vi "UMLEditor_GetP.vi"(8 "error in (no error)":errorcluster, 10 "GetProjectRefByName/or Ref":variant) -> (0 "error out":errorcluster, 1 "j":i32, 2 "i":i32, 3 "ClassesNamesAndPaths":T1[](array[typedef]), 4 "A":i32, 6 "B":i32)   [LabVIEW 2012]
uses:
  <resource>/Framework/Providers/Open_GDS/ClassProviders/Common/CommonVIs/CommonVIs_ClassNamePathType.ctl
  <resource>/Framework/Providers/Open_GDS/ClassProviders/Common/LvClass_class/GDSLvClass_ClassTypeSettingNames.ctl
  <resource>/Framework/Providers/Open_GDS/ClassProviders/Provider_EndevoGOOP300/EndevoProviderName.ctl
  <resource>/Framework/Providers/Open_GDS/ClassProviders/Provider_EndevoGOOP400/EndevoG4ProviderName.ctl
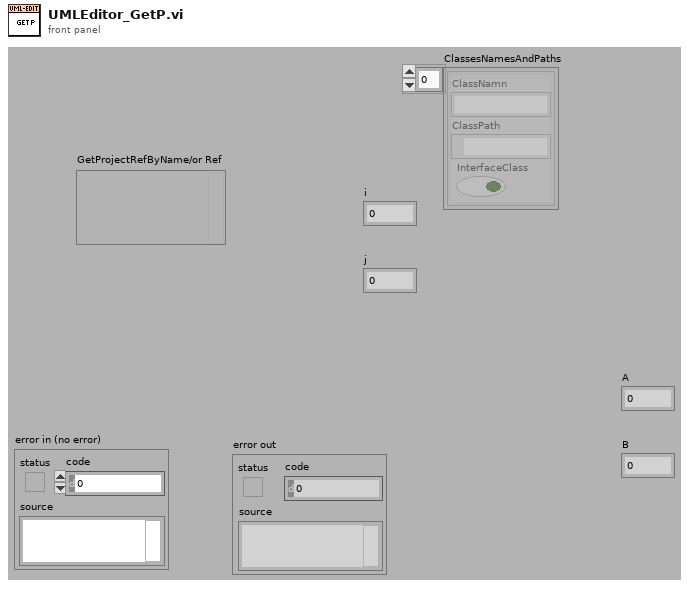
[diagram p1: front panel]
types:
  T1 = typedef "CommonVIs_ClassNamePathType.ctl" = cluster{"ClassNamn":string, "ClassPath":path, "InterfaceClass":bool}
  T2 = typedef "EndevoG4ProviderName.ctl" = enum16{"EndevoGOOP400"}
  T3 = typedef "EndevoProviderName.ctl" = enum16{"EndevoGOOP300"}
  T4 = typedef "GDSLvClass_ClassTypeSettingNames.ctl" = enum16{"EndevoGOOP_ClassProvider", "EndevoGOOP_TemplateUsed", "EndevoGOOP_TemplateVersion", "EndevoGOOP_PlugIns", "EndevoGOOP_ConnectorPanePattern"}
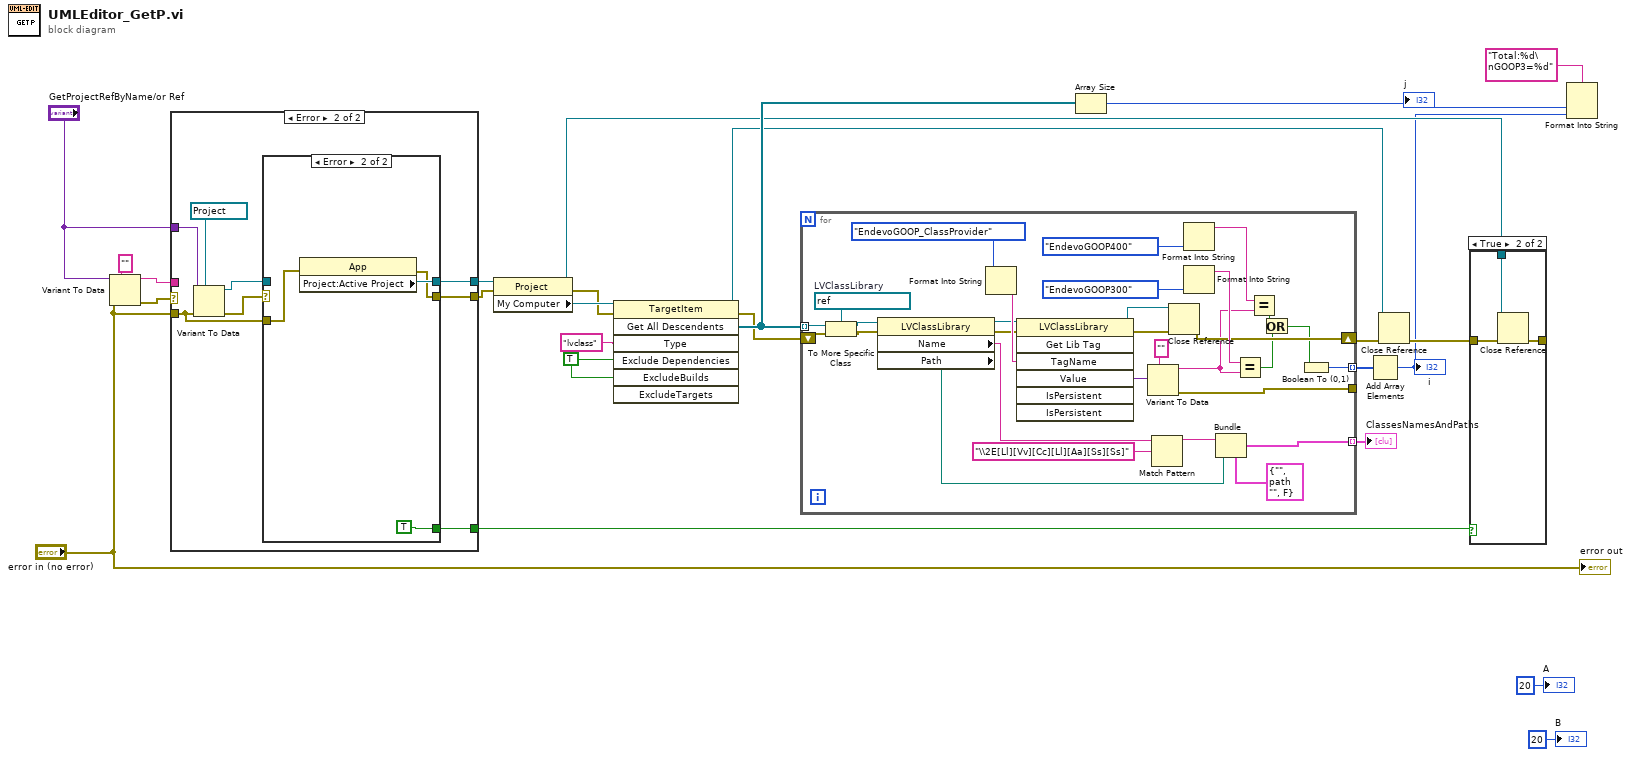
[diagram p0: block diagram]
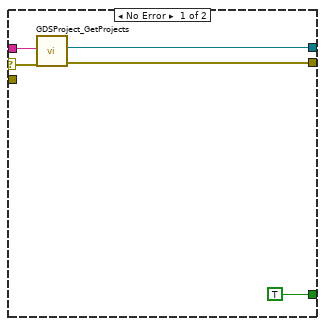
[diagram p3: hidden frame]
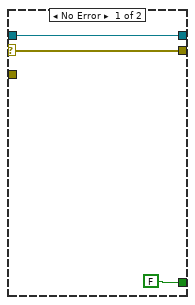
[diagram p4: hidden frame]
diagram:
  w4 = TRUE ("ExcludeDependencies")
  n1 = Variant To Data(error in="error in (no error)", type="", Variant="GetProjectRefByName/or Ref") -> (data=w15:string, error out=w14:errorcluster)
  n2 = case shown="Error" w14 {
    selector: w14 -> [w27 _]
    tunnel: [w30 w34] -> w25
    tunnel: [w29 w33] -> w21
    tunnel: w15 -> [w28 _]
    tunnel: "error in (no error)" -> [_ w32]
    tunnel: "GetProjectRefByName/or Ref" -> [_ w37]
    tunnel: [TRUE w31] -> w5
    frame No Error {
      n3 = call <resource>:"GDSProject_GetProjects.vi"("GetProjectRefByName"=w28, "error in (no error)"=w27) -> ("Project Refnum"=w30:refnum<vi>, "error out"=w29:errorcluster)  [unwired: 1 in, 15 out]
    }
    frame Error {
      n4 = Variant To Data(error in=w32, type=refnum<vi> refnum ("Project Refnum"), Variant=w37) -> (data=w35:refnum<vi>, error out=w36:errorcluster)
      n5 = case shown="Error" w36 {
        selector: w36 -> [w40 _]
        tunnel: w35 -> [w41 _]
        tunnel: [w41 w45] -> w34
        tunnel: [w40 w43] -> w33
        tunnel: w32 -> [_ w44]
        tunnel: [FALSE TRUE] -> w31
        frame No Error {
        }
        frame Error {
          n6 = property class="App"(error in=w44) -> (error out=w43:errorcluster, "Project:Active Project"=w45:refnum<vi>)  [unwired: 1 in, 1 out]
        }
      }
    }
  }
  n7 = property class="Project"(reference=w25, error in=w21) -> (reference out=w17:refnum<vi>, error out=w12:errorcluster, "My Computer"=w24:refnum<vi>)
  n8 = invoke class="TargetItem" method="Get All Descendents"(reference=w24, error in=w12, "Type"="lvclass", "Exclude Dependencies"=w4, "ExcludeBuilds"=w4) -> (reference out=w18:refnum<vi>, error out=w11:errorcluster, "All Descendents"=w20:refnum<vi>[])  [unwired: 2 in, 4 out]
  n9 = for {
    tunnel: w20 -> [w70] mode=indexing
    tunnel: [w67] -> w22 mode=indexing
    shift-right: [w63] -> w19
    shift-left: w11 -> [w66]
    tunnel: [w62] -> _
    tunnel: [w53] -> w3 mode=indexing
    w75 = refnum<vi> refnum  # LVClassLibrary
    n10 = To More Specific Class(target class=w75, reference=w70, error in=w66) -> (specific class reference=w61:refnum<vi>, error out=w60:errorcluster)
    n11 = property class="LVClassLibrary"(reference=w61, error in=w60) -> (reference out=w59:refnum<vi>, error out=w58:errorcluster, "Name"=w57:string, "Path"=w54:path)
    n12 = Format Into String(GDSLvClass_ClassTypeSettingNames."EndevoGOOP_ClassProvider" ("ClassTypeSettingNames")) -> (resulting string=w72:string)  [unwired: 3 in, 1 out]
    n13 = invoke class="LVClassLibrary" method="Get Lib Tag"(reference=w59, error in=w58, "TagName"=w72) -> (reference out=w65:refnum<vi>, error out=w64:errorcluster, "Value"=w74:variant)  [unwired: 4 in, 4 out]
    n14 = Variant To Data(type="", Variant=w74) -> (data=w51:string, error out=w62:errorcluster)  [unwired: 1 in]
    n15 = Match Pattern(string=w57, regular expression="\\2E[Ll][Vv][Cc][Ll][Aa][Ss][Ss]") -> (before substring=w55:string)  [unwired: 4 out]
    n16 = Close Reference(reference=w65, error in (no error)=w64) -> (error out=w63:errorcluster)
    n17 = Format Into String(EndevoG4ProviderName."EndevoGOOP400" ("ProviderName")) -> (resulting string=w50:string)  [unwired: 3 in, 1 out]
    n18 = Format Into String(EndevoProviderName."EndevoGOOP300" ("ProviderName")) -> (resulting string=w68:string)  [unwired: 3 in, 1 out]
    n19 = Bundle(cluster=T1 {"ClassNamn"="", "ClassPath"=path "", "InterfaceClass"=FALSE} ("Cluster"), "ClassNamn"=w55, "ClassPath"=w54) -> (w53:T1)  [unwired: 1 in]
    n20 = Equal?(x=w68, y=w51) -> (x = y?=w48:bool)
    n21 = Equal?(x=w50, y=w51) -> (x = y?=w49:bool)
    n22 = Or(x=w49, y=w48) -> (x .or. y?=w47:bool)
    n23 = Boolean To (0,1)(Boolean=w47) -> (0, 1=w67:i16)
  }
  "ClassesNamesAndPaths" <- w3
  n24 = Array Size(array=w20) -> (size(s)=w10:i32)
  "j" <- w10
  n25 = Add Array Elements(numeric array=w22) -> (sum=w8:i16)
  "i" <- w8
  n26 = Close Reference(reference=w18, error in (no error)=w19) -> (error out=w13:errorcluster)
  n27 = case shown="True" w5 {
    tunnel: w13 -> [_ w78]
    tunnel: w17 -> [_ w77]
    tunnel: [_ w76] -> _
    frame False {
    }
    frame True {
      n28 = Close Reference(reference=w77, error in (no error)=w78) -> (error out=w76:errorcluster)
    }
  }
  n29 = Format Into String(format string="Total:%d\nGOOP3=%d", w10, w8) -> ()  [unwired: 2 in, 2 out]
  "error out" <- "error in (no error)"
  "A" <- 20 ("A")
  "B" <- 20 ("B")
